vi "Determine Value Type.vi"(8 "error in (no error)":errorcluster, 11 "Composed Column Factory in":refnum<class "Composed Column Factory.lvclass">) -> (0 "error out":errorcluster, 2 "Value Type":refnum<class "Value Type.lvclass">, 3 "Composed Column Factory out":refnum<class "Composed Column Factory.lvclass">)   [LabVIEW 2020, in "Composed Columns.lvlib" / "Composed Column Factory.lvclass"]
uses:
  Composed Column Factory.lvclass
  Value Type/Value Type.lvclass
  Composed Column Factory.lvclass/Composed Column Factory.ctl
  String Value/String Value.lvclass
  C:/Users/User/Desktop/Raman Program/Database OOP/source/Database OOP/Column Libraries/Value Type/Value Type.lvclass
  Numeric Value/Numeric Value.lvclass
  Timestamp Value/Timestamp Value.lvclass
  Basic Columns/Column Configuration/Basic Column Configuration Class/Column Configuration.lvclass
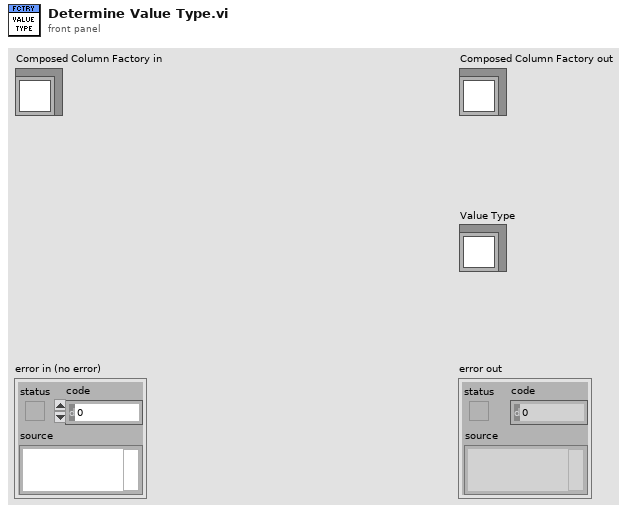
[diagram p1: front panel]
types:
  T1 = typedef "Database Interfaces.lvlib/Database data type.ctl" = enum16{"Undefined", "String", "Long (I32)", "Single (SGL)", "Double (DBL)", "Date/Time", "Binary"}
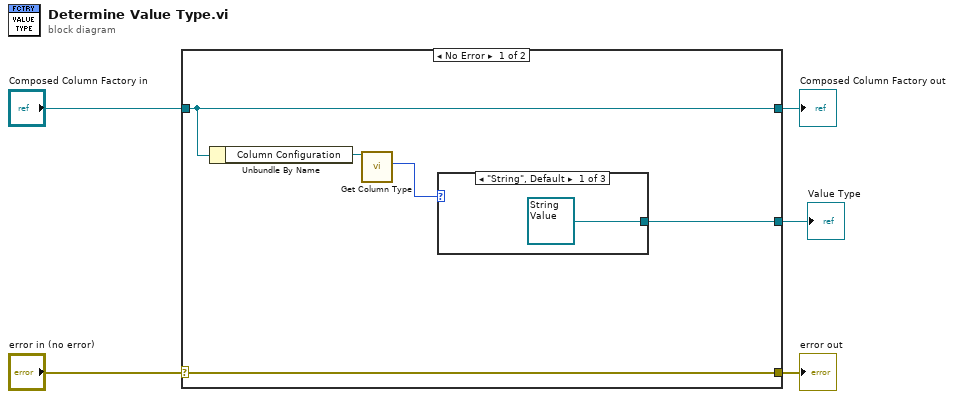
[diagram p0: block diagram]
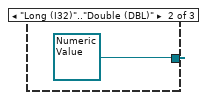
[diagram p2: hidden frame]
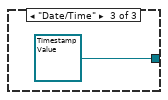
[diagram p3: hidden frame]
diagram:
  n1 = case shown="No Error" "error in (no error)" {
    selector: "error in (no error)" -> [w10 w15]
    tunnel: [w10 w15] -> w4
    tunnel: [w7 w14] -> w2
    tunnel: "Composed Column Factory in" -> [w7 w14]
    tunnel: [w9 _] -> w1
    frame No Error {
      n2 = Unbundle By Name(w7) -> ("Column Configuration"=w8:refnum<class "Column Configuration.lvclass">)
      n3 = call-dynamic "Get Column Type.vi"("Basic Column Configuration in"=w8) -> ("Column Type"=w6:T1)  [unwired: 8 in, 2 out]
      n4 = case shown="\"String\", Default" w6 {
        tunnel: [refnum<class "String Value.lvclass"> refnum ("Composed Columns.lvlib:String Value.lvclass") refnum<class "Numeric Value.lvclass"> refnum ("Composed Columns.lvlib:Numeric Value.lvclass") refnum<class "Timestamp Value.lvclass"> refnum ("Composed Columns.lvlib:Timestamp Value.lvclass")] -> w9
        frame "String", Default {
        }
        frame "Long (I32)".."Double (DBL)" {
        }
        frame "Date/Time" {
        }
      }
    }
    frame Error {
    }
  }
  "error out" <- w4
  "Composed Column Factory out" <- w2
  "Value Type" <- w1
